vi "Construct.vi"(1 "Rectangle Shape in":refnum<class "RectangleShape.lvclass">) -> (0 "Rect Collider out":refnum<class "Rect Collider.lvclass">)   [LabVIEW 2022 SP3, in "Rect Collider.lvclass"]
uses:
  Rect Collider.lvclass
  Rect Collider.lvclass/Rect Collider.ctl
  Shapes/RectangleShape/RectangleShape.lvclass
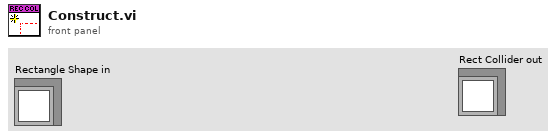
[diagram p1: front panel]
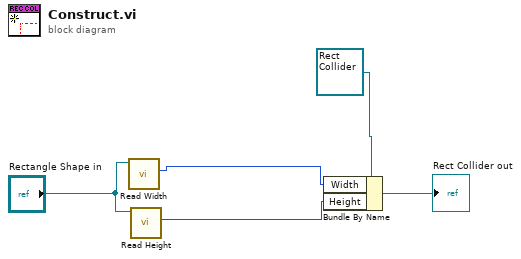
[diagram p0: block diagram]
diagram:
  n1 = call "Read Width.vi"("RectangleShape in"="Rectangle Shape in") -> ("Width"=w3:i16)  [unwired: 8 in, 2 out]
  n2 = call "Read Height.vi"("RectangleShape in"="Rectangle Shape in") -> ("Height"=w2:i16)  [unwired: 8 in, 2 out]
  n3 = Bundle By Name(cluster=refnum<class "Rect Collider.lvclass"> refnum ("Rect Collider.lvclass"), "Width"=w3, "Height"=w2) -> (→"Rect Collider out":refnum<class "Rect Collider.lvclass">)
